vi "Set Instrument.vi"(10 "HAL.lvlib:Instrument":refnum<class "Instrument.lvclass">, 11 "Virtual Instrument in":refnum<class "Virtual Instrument.lvclass">) -> (3 "Virtual Instrument out":refnum<class "Virtual Instrument.lvclass">)   [LabVIEW 2023, in "HAL.lvlib" / "Virtual Instrument.lvclass"]
uses:
  Virtual Instrument.lvclass
  Virtual Instrument.lvclass/Virtual Instrument.ctl
  Instrument/Instrument.lvclass
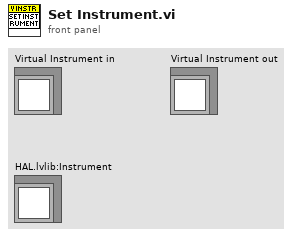
[diagram p1: front panel]
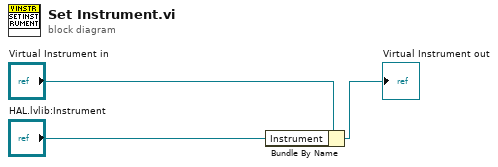
[diagram p0: block diagram]
diagram:
  n1 = Bundle By Name(cluster="Virtual Instrument in", "Instrument"="HAL.lvlib:Instrument") -> (→"Virtual Instrument out":refnum<class "Virtual Instrument.lvclass">)
